vi "Get Item Cell Strings.vi"(0 "Tree Reference In":refnum<vi>, 1 "Tag (Current)":string, 5 "error in (no error)":errorcluster, 9 "# of Columns":u8) -> (14 "Tree Reference Out":refnum<vi>, 15 "Duplicate Tag":string, 16 "Left Cell String":string, 17 "Cell Strings":string[](array[string]), 19 "error out":errorcluster)   [LabVIEW 2015, in "QuickVIew.lvlib"]
doc: "Get all the cell strings for the given tag - if empty tag - it considers the current tag\nIf # of columns is 0, Get all the text until finding an empty strings. Else read the needed number of columns. Give the left most cell string information separately\nTLB Prime - Application Template 1.3.0.24\nNorm Kirchner, NI Systems Engineering - NI\nCopyright (c) 2014, NI"
uses:
  QuickVIew.lvlib
panel:
  # "VI INPUTS"
  # "VI LOCALS"
  # "VI OUTPUTS"
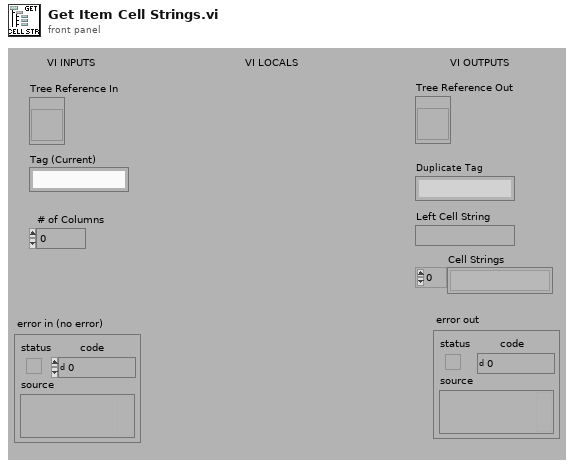
[diagram p1: front panel]
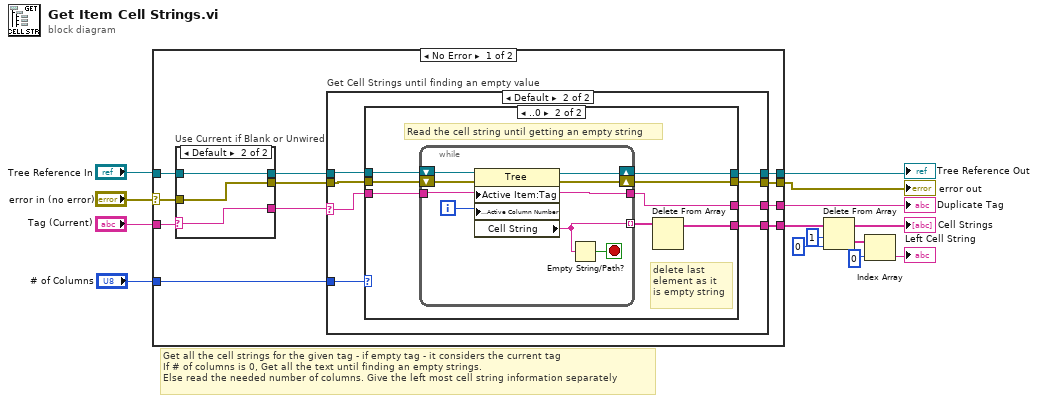
[diagram p0: block diagram]
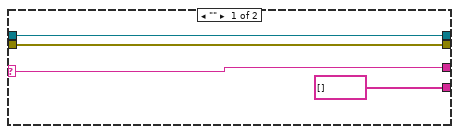
[diagram p2: hidden frame]
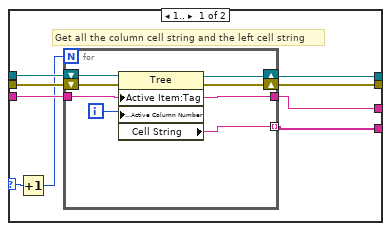
[diagram p3: hidden frame]
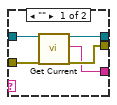
[diagram p4: hidden frame]
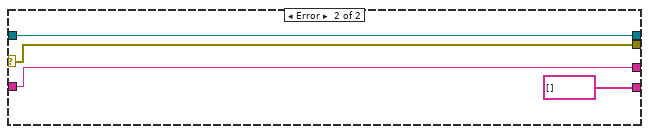
[diagram p5: hidden frame]
diagram:
  # "Get all the cell strings for the given tag - if empty tag - it considers the current tag\nIf # of columns is 0, Get all the text until finding an empty strings. \nElse read the needed number of columns. Give the left most cell string information separately"
  n1 = case shown="No Error" "error in (no error)" {
    selector: "error in (no error)" -> [w24 w80]
    tunnel: "Tree Reference In" -> [w25 w81]
    tunnel: [w23 w81] -> w12
    tunnel: [w22 w80] -> w11
    tunnel: [w18 w79] -> w9
    tunnel: "Tag (Current)" -> [w17 w79]
    tunnel: [w16 string[] []] -> w7
    tunnel: "# of Columns" -> [w15 _]
    frame No Error {
      n2 = case "Use Current if Blank or Unwired" shown="Default" w17 {
        selector: w17 -> [_ w75]
        tunnel: [w73 w77] -> w21
        tunnel: w25 -> [w74 w77]
        tunnel: [w72 w76] -> w20
        tunnel: w24 -> [w71 w76]
        tunnel: [w70 w75] -> w19
        frame "" {
          n3 = call "Get Current.vi"("Tree Reference In"=w74, "error in (no error)"=w71) -> ("Tree Reference Out"=w73:refnum<vi>, "Current Tag"=w70:string, "error out"=w72:errorcluster)  [unwired: 14 in, 1 out]
        }
        frame Default {
        }
      }
      n4 = case "Get Cell Strings until finding an empty value" shown="Default" w19 {
        selector: w19 -> [w27 w33]
        tunnel: [w29 w35] -> w23
        tunnel: [w28 w34] -> w22
        tunnel: w21 -> [w29 w37]
        tunnel: w20 -> [w28 w36]
        tunnel: [w27 w32] -> w18
        tunnel: [string[] [] w31] -> w16
        tunnel: w15 -> [_ w30]
        frame "" {
        }
        frame Default {
          n5 = case shown="..0" w30 {
            selector: w30 -> [w40 _]
            tunnel: w37 -> [w46 w61]
            tunnel: w36 -> [w45 w60]
            tunnel: [w44 w59] -> w35
            tunnel: [w43 w58] -> w34
            tunnel: w33 -> [w42 w57]
            tunnel: [w41 w56] -> w32
            tunnel: [w39 w54] -> w31
            frame 1.. {
              # "Get all the column cell string and the left cell string"
              n6 = Increment(x=w40) -> (x+1=w38:u8)
              n7 = for {
                N: w38 -> [_]
                tunnel: w42 -> [w49]
                shift-right: [w51] -> w44
                shift-left: w46 -> [w53]
                shift-right: [w50] -> w43
                shift-left: w45 -> [w52]
                tunnel: [w48] -> w39 mode=indexing
                tunnel: [w49] -> w41
                i -> [w47]
                n8 = property class="Tree"(reference=w53, error in=w52, "Active Item:Tag"=w49, "Active Cell:Active Column Number"=w47) -> (reference out=w51:refnum<vi>, error out=w50:errorcluster, "Cell String"=w48:string)
              }
            }
            frame ..0 {
              # "Read the cell string until getting an empty string"
              # "delete last\nelement as it \nis empty string"
              n9 = while {
                tunnel: w57 -> [w65]
                shift-right: [w67] -> w59
                shift-left: w61 -> [w69]
                shift-right: [w66] -> w58
                shift-left: w60 -> [w68]
                tunnel: [w64] -> w55 mode=indexing
                tunnel: [w65] -> w56
                i -> [w62]
                stop <- w63 stop-if-true
                n10 = property class="Tree"(reference=w69, error in=w68, "Active Item:Tag"=w65, "Active Cell:Active Column Number"=w62) -> (reference out=w67:refnum<vi>, error out=w66:errorcluster, "Cell String"=w64:string)
                n11 = Empty String/Path?(string/path=w64) -> (empty?=w63:bool)
              }
              n12 = Delete From Array(array=w55) -> (array with subset deleted=w54:string[])  [unwired: 2 in, 1 out]
            }
          }
        }
      }
    }
    frame Error {
    }
  }
  "error out" <- w11
  "Tree Reference Out" <- w12
  "Duplicate Tag" <- w9
  n13 = Delete From Array(array=w7, length=1, index=0) -> (deleted portion=w4:string[], array with subset deleted=→"Cell Strings":string[])
  n14 = Index Array(array=w4, index=0) -> (element=→"Left Cell String":string)
